vi "MH_Count_Records_and_TT.vi"(8 "error in (no error)":errorcluster caption="entrée d'erreur (pas d'erreur)", 11 "RecBuffer":u32[](array[numeric])) -> (0 "error out":errorcluster caption="sortie d'erreur", 3 "Photon Counts":u32)   [LabVIEW 2019]
uses:
  4c953fbe-1250-4e84-8fbe-ba1aaf1de92e.vi
  df5dff5d-21f2-4b0b-b63d-1d0949650618.vi
panel:
  in  "oflcorr_In":u64
  out "oflcorr_out":u64
  out "BinTime Out":u64
  in  "BinTime":u64
  out "TBinIdxOut":i32 caption="indice"
  in  "TBinIdx":i32 caption="indice"
  in  "Ch1TTrace In":u64[](array[numeric])
  out "Ch1TTrace":u64[](array[numeric])
  in  "TimeBinWidth":u64
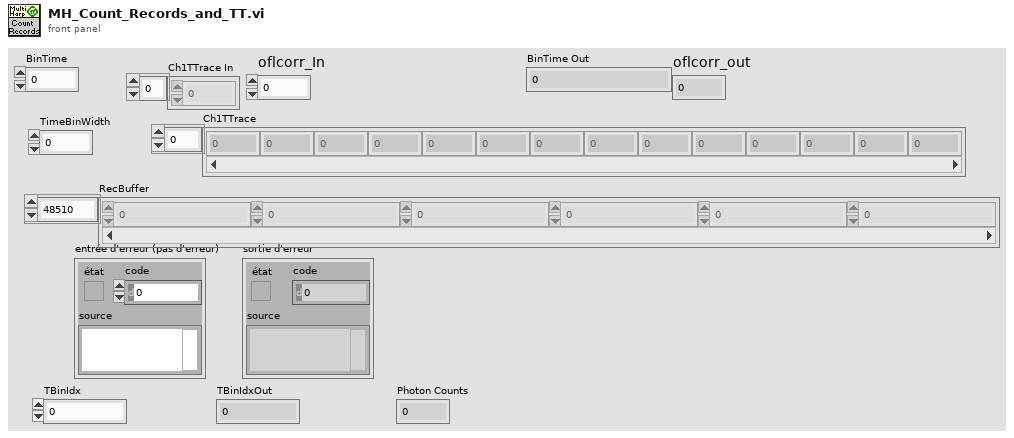
[diagram p1: front panel]
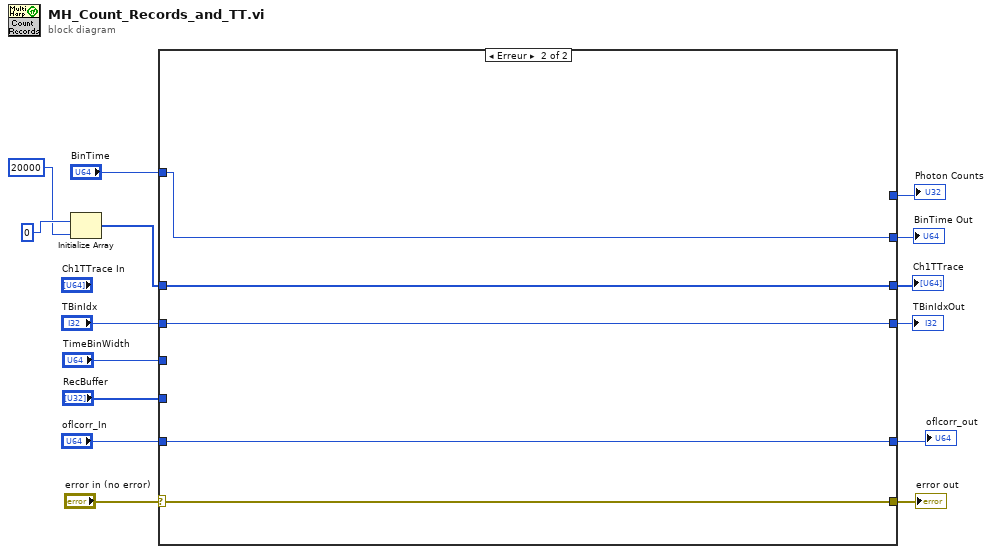
[diagram p0: block diagram]
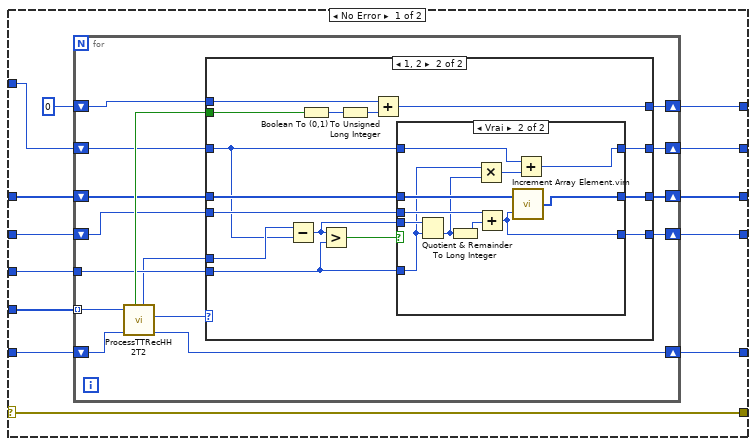
[diagram p2: hidden frame]
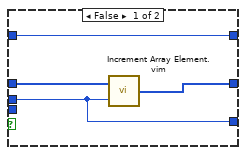
[diagram p4: hidden frame]
diagram:
  n1 = Initialize Array(u64 0 ("Ch1TTrace In"), 20000 ("taille de la dimension")) -> (w7:u64[])
  n2 = case shown="Erreur" "error in (no error)" {
    selector: "error in (no error)" -> [w28 w82]
    tunnel: [w28 w82] -> w12
    tunnel: "RecBuffer" -> [w27 _]
    tunnel: [w25 _] -> w13
    tunnel: "TimeBinWidth" -> [w24 _]
    tunnel: w7 -> [w23 w81]
    tunnel: "TBinIdx" -> [w22 w80]
    tunnel: [w21 w80] -> w9
    tunnel: [w20 w81] -> w8
    tunnel: "BinTime" -> [w19 w79]
    tunnel: [w18 w79] -> w3
    tunnel: [w17 w78] -> w2
    tunnel: "oflcorr_In" -> [w16 w78]
    frame No Error {
      n3 = for {
        tunnel: w27 -> [w43] mode=indexing
        shift-right: [w41] -> w25
        shift-left: u32 0 -> [w29]
        shift-right: [w40] -> w17
        shift-left: w16 -> [w39]
        shift-right: [w33] -> w18
        shift-left: w19 -> [w31]
        tunnel: w24 -> [w34]
        shift-right: [w37] -> w20
        shift-left: w23 -> [w38]
        shift-right: [w35] -> w21
        shift-left: w22 -> [w36]
        n4 = call <userlib>:"ProcessTTRecHH2T2.vi"("oflcorr_in"=w39, "rawbits"=w43) -> ("oflcorr_out"=w40:u64, "channel"=w30:u32, "truetime"=w32:u64, "is_photon"=w42:bool)  [unwired: 4 in, 2 out]
        n5 = case shown="1, 2" w30 {
          tunnel: w42 -> [_ w60]
          tunnel: [w47 w59] -> w41
          tunnel: w29 -> [w47 w58]
          tunnel: w38 -> [w45 w56]
          tunnel: [w45 w55] -> w37
          tunnel: w36 -> [w44 w54]
          tunnel: [w44 w53] -> w35
          tunnel: w34 -> [_ w51]
          tunnel: [w46 w50] -> w33
          tunnel: w32 -> [_ w49]
          tunnel: w31 -> [w46 w48]
          frame 0, Default {
          }
          frame 1, 2 {
            n6 = Subtract(x=w49, y=w48) -> (x-y=w52:u64)
            n7 = Boolean To (0,1)(Boolean=w60) -> (0, 1=w62:i16)
            n8 = Greater?(x=w52, y=w51) -> (0:w57:bool)
            n9 = To Unsigned Long Integer(number=w62) -> (unsigned 32bit integer=w61:u32)
            n10 = Add(x=w58, y=w61) -> (x+y=w59:u32)
            n11 = case shown="Vrai" w57 {
              tunnel: w56 -> [w66 w77]
              tunnel: [w65 w73] -> w55
              tunnel: w54 -> [w64 w75]
              tunnel: [w64 w74] -> w53
              tunnel: w52 -> [_ w76]
              tunnel: w51 -> [_ w71]
              tunnel: [w63 w69] -> w50
              tunnel: w48 -> [w63 w67]
              frame False {
                n12 = call "Increment Array Element.vim"("index"=w64, "array in"=w66) -> ("array out"=w65:u64[])
              }
              frame True {
                n13 = Quotient & Remainder(x=w76, y=w71) -> (floor(x/y)=w70:u64)  [unwired: 1 out]
                n14 = To Long Integer(number=w70) -> (32bit integer=w72:i32)
                n15 = Multiply(x=w71, y=w70) -> (x*y=w68:u64)
                n16 = Add(x=w75, y=w72) -> (x+y=w74:i32)
                n17 = call "Increment Array Element.vim"("index"=w74, "array in"=w77) -> ("array out"=w73:u64[])
                n18 = Add(x=w67, y=w68) -> (x+y=w69:u64)
              }
            }
          }
        }
      }
    }
    frame Error {
    }
  }
  "error out" <- w12
  "Photon Counts" <- w13
  "Ch1TTrace" <- w8
  "TBinIdxOut" <- w9
  "BinTime Out" <- w3
  "oflcorr_out" <- w2
